vi "步响应_找到所有峰.vi"(0 "行程 in":dbl[](array[numeric]), 1 "nb_of_peaks":dbl=10.0 format="%#_13g", 2 "X_peak_start":dbl, 3 "step_peak":dbl, 4 "（要求）连续大于0的次数":dbl=10.0 format="%#_13g") -> (5 "行程 out":dbl[](array[numeric]), 6 "X_Peaks":dbl[](array[numeric]), 7 "Y_Peaks":dbl[](array[numeric]))   [LabVIEW 2013]
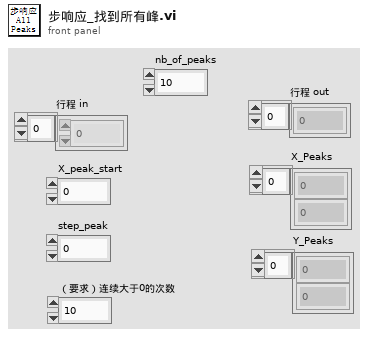
[diagram p1: front panel]
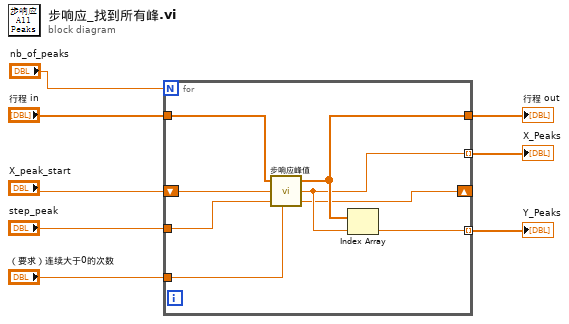
[diagram p0: block diagram]
diagram:
  n1 = for {
    N: "nb_of_peaks" -> [_]
    tunnel: "step_peak" -> [w16]
    tunnel: "行程 in" -> [w14]
    shift-right: [w10] -> _
    shift-left: "X_peak_start" -> [w15]
    tunnel: [w13] -> w5
    tunnel: [w12] -> w4 mode=indexing
    tunnel: [w11] -> w3 mode=indexing
    tunnel: "（要求）连续大于0的次数" -> [w9]
    n2 = call "步响应峰值.vi"("行程 in"=w14, "X_start"=w15, "peak_step"=w16, "（要求）连续大于0的次数"=w9) -> ("行程 out"=w13:dbl[], "X_value"=w12:dbl, "X_value_next"=w10:dbl)  [unwired: 1 in]
    n3 = Index Array(array=w13, index=w12) -> (element=w11:dbl)
  }
  "行程 out" <- w5
  "X_Peaks" <- w4
  "Y_Peaks" <- w3
